vi "Loop.vi"(0 "Input parameters":T2={"Measurement type"=enum."Debug", "Sensor type"=enum."HPK_8in_256", "Identifier"="test.txt", "Open after execution?"=FALSE, "Plot after execution?"=FALSE, "Display channel"=0, "Voltage Delay (s)"=0.5, "Switch Delay (s)"=0.01, "VISA resource name source"="", "VISA resource name DMM"="", "VISA resource name LCR"="", "Compliance  Level (A)"=10.0, "Voltage Limit (V)"=1000.0, "Data storage location"="", "Scan voltages"="", "Use source as DMM?"=FALSE, "LCR signal frequenzy (Hz)"=10.0, "DMM device"=enum."Keithley2001", "Sampling number"=1, "Use env. sensors on"=enum."Sensirion sht1x/7x", "Switchboard Handle"=0, "Use Switchboard"=FALSE, "LCR signal voltage (V)"=10000.0, "Repeat"=1, "Scan voltages IV"="", "Scan voltages CV"="", "Hex pad numbers?"=FALSE, "Set measurement type"=enum."Debug", "Custom pad scan"="", "IV voltage Delay (s)"=0.5, "CV voltage Delay (s)"=0.5, "Needle measurement?"=FALSE, "Comments"="test.txt", "LCR signal frequenzy (kHz)"=10.0, "Compliance  Level (uA)"=10.0, "Open Correction Array"=array2304x3[6912 elements], "Current set voltage"=0.0, "Last set voltage"=0.0, "Current channel"=0, "Last OpenCorrection index"=-1, "Total curr/vltg every x steps"=10, "Current channel iteration"=0, "No CV corrections"=FALSE, "Mapfile"="", "Corrfile"="", "Invert polarity"=FALSE} {"Last set voltage" format="%#_13g"; "Current set voltage" format="%#_13g"; "CV voltage Delay (s)" format="%#_13g"; "IV voltage Delay (s)" format="%#_13g"; "Voltage Limit (V)" format="%#_13g"; "Voltage Delay (s)" format="%#_13g"; "Switch Delay (s)" format="%#_13g"}, 5 "Dynamic data":T4, 7 "Front_panel_refs":T1, 11 "error in (no error)":errorcluster, 12 "Environmental data":T3) -> (4 "Input parameters out":T2={"Measurement type"=enum."Debug", "Sensor type"=enum."HPK_8in_256", "Identifier"="test.txt", "Open after execution?"=FALSE, "Plot after execution?"=FALSE, "Display channel"=0, "Voltage Delay (s)"=0.5, "Switch Delay (s)"=0.01, "VISA resource name source"="", "VISA resource name DMM"="", "VISA resource name LCR"="", "Compliance  Level (A)"=10.0, "Voltage Limit (V)"=1000.0, "Data storage location"="", "Scan voltages"="", "Use source as DMM?"=FALSE, "LCR signal frequenzy (Hz)"=10.0, "DMM device"=enum."Keithley2001", "Sampling number"=1, "Use env. sensors on"=enum."Sensirion sht1x/7x", "Switchboard Handle"=0, "Use Switchboard"=FALSE, "LCR signal voltage (V)"=10000.0, "Repeat"=1, "Scan voltages IV"="", "Scan voltages CV"="", "Hex pad numbers?"=FALSE, "Set measurement type"=enum."Debug", "Custom pad scan"="", "IV voltage Delay (s)"=0.5, "CV voltage Delay (s)"=0.5, "Needle measurement?"=FALSE, "Comments"="test.txt", "LCR signal frequenzy (kHz)"=10.0, "Compliance  Level (uA)"=10.0, "Open Correction Array"=array2304x3[6912 elements], "Current set voltage"=0.0, "Last set voltage"=0.0, "Current channel"=0, "Last OpenCorrection index"=-1, "Total curr/vltg every x steps"=10, "Current channel iteration"=0, "No CV corrections"=FALSE, "Mapfile"="", "Corrfile"="", "Invert polarity"=FALSE} {"Last set voltage" format="%#_13g"; "Current set voltage" format="%#_13g"; "CV voltage Delay (s)" format="%#_13g"; "IV voltage Delay (s)" format="%#_13g"; "Voltage Limit (V)" format="%#_13g"; "Voltage Delay (s)" format="%#_13g"; "Switch Delay (s)" format="%#_13g"}, 6 "Dynamic data out":T4, 8 "Front_panel_refs out":T1, 15 "error out":errorcluster)   [LabVIEW 2016]
uses:
  Input_parameters.ctl
  Dynamic_data.ctl
  <extravilib>/ChannelInstances/Tag-t'Env_data.ctl'/))Channel.ctl
  Env_data.ctl
  Front_panel_refs.ctl
  Live_data.ctl
  <extravilib>/ChannelInstances/Tag-t'Env_data.ctl'/Read With Abort.vi
  <extravilib>/ChannelInstances/Tag-t'Env_data.ctl'/Endpoint.vi
  <extravilib>/ChannelInstances/Tag-t'Env_data.ctl'.lvlib
panel:
  out "Input parameters display":T2={"Measurement type"=enum."Debug", "Sensor type"=enum."HPK_8in_256", "Identifier"="test.txt", "Open after execution?"=FALSE, "Plot after execution?"=FALSE, "Display channel"=0, "Voltage Delay (s)"=0.5, "Switch Delay (s)"=0.01, "VISA resource name source"="", "VISA resource name DMM"="", "VISA resource name LCR"="", "Compliance  Level (A)"=10.0, "Voltage Limit (V)"=1000.0, "Data storage location"="", "Scan voltages"="", "Use source as DMM?"=FALSE, "LCR signal frequenzy (Hz)"=10.0, "DMM device"=enum."Keithley2001", "Sampling number"=1, "Use env. sensors on"=enum."Sensirion sht1x/7x", "Switchboard Handle"=0, "Use Switchboard"=FALSE, "LCR signal voltage (V)"=10000.0, "Repeat"=1, "Scan voltages IV"="", "Scan voltages CV"="", "Hex pad numbers?"=FALSE, "Set measurement type"=enum."Debug", "Custom pad scan"="", "IV voltage Delay (s)"=0.5, "CV voltage Delay (s)"=0.5, "Needle measurement?"=FALSE, "Comments"="test.txt", "LCR signal frequenzy (kHz)"=10.0, "Compliance  Level (uA)"=10.0, "Open Correction Array"=array2304x3[6912 elements], "Current set voltage"=0.0, "Last set voltage"=0.0, "Current channel"=0, "Last OpenCorrection index"=-1, "Total curr/vltg every x steps"=10, "Current channel iteration"=0, "No CV corrections"=FALSE, "Mapfile"="", "Corrfile"="", "Invert polarity"=FALSE} {"Last set voltage" format="%#_13g"; "Current set voltage" format="%#_13g"; "CV voltage Delay (s)" format="%#_13g"; "IV voltage Delay (s)" format="%#_13g"; "Voltage Limit (V)" format="%#_13g"; "Voltage Delay (s)" format="%#_13g"; "Switch Delay (s)" format="%#_13g"}
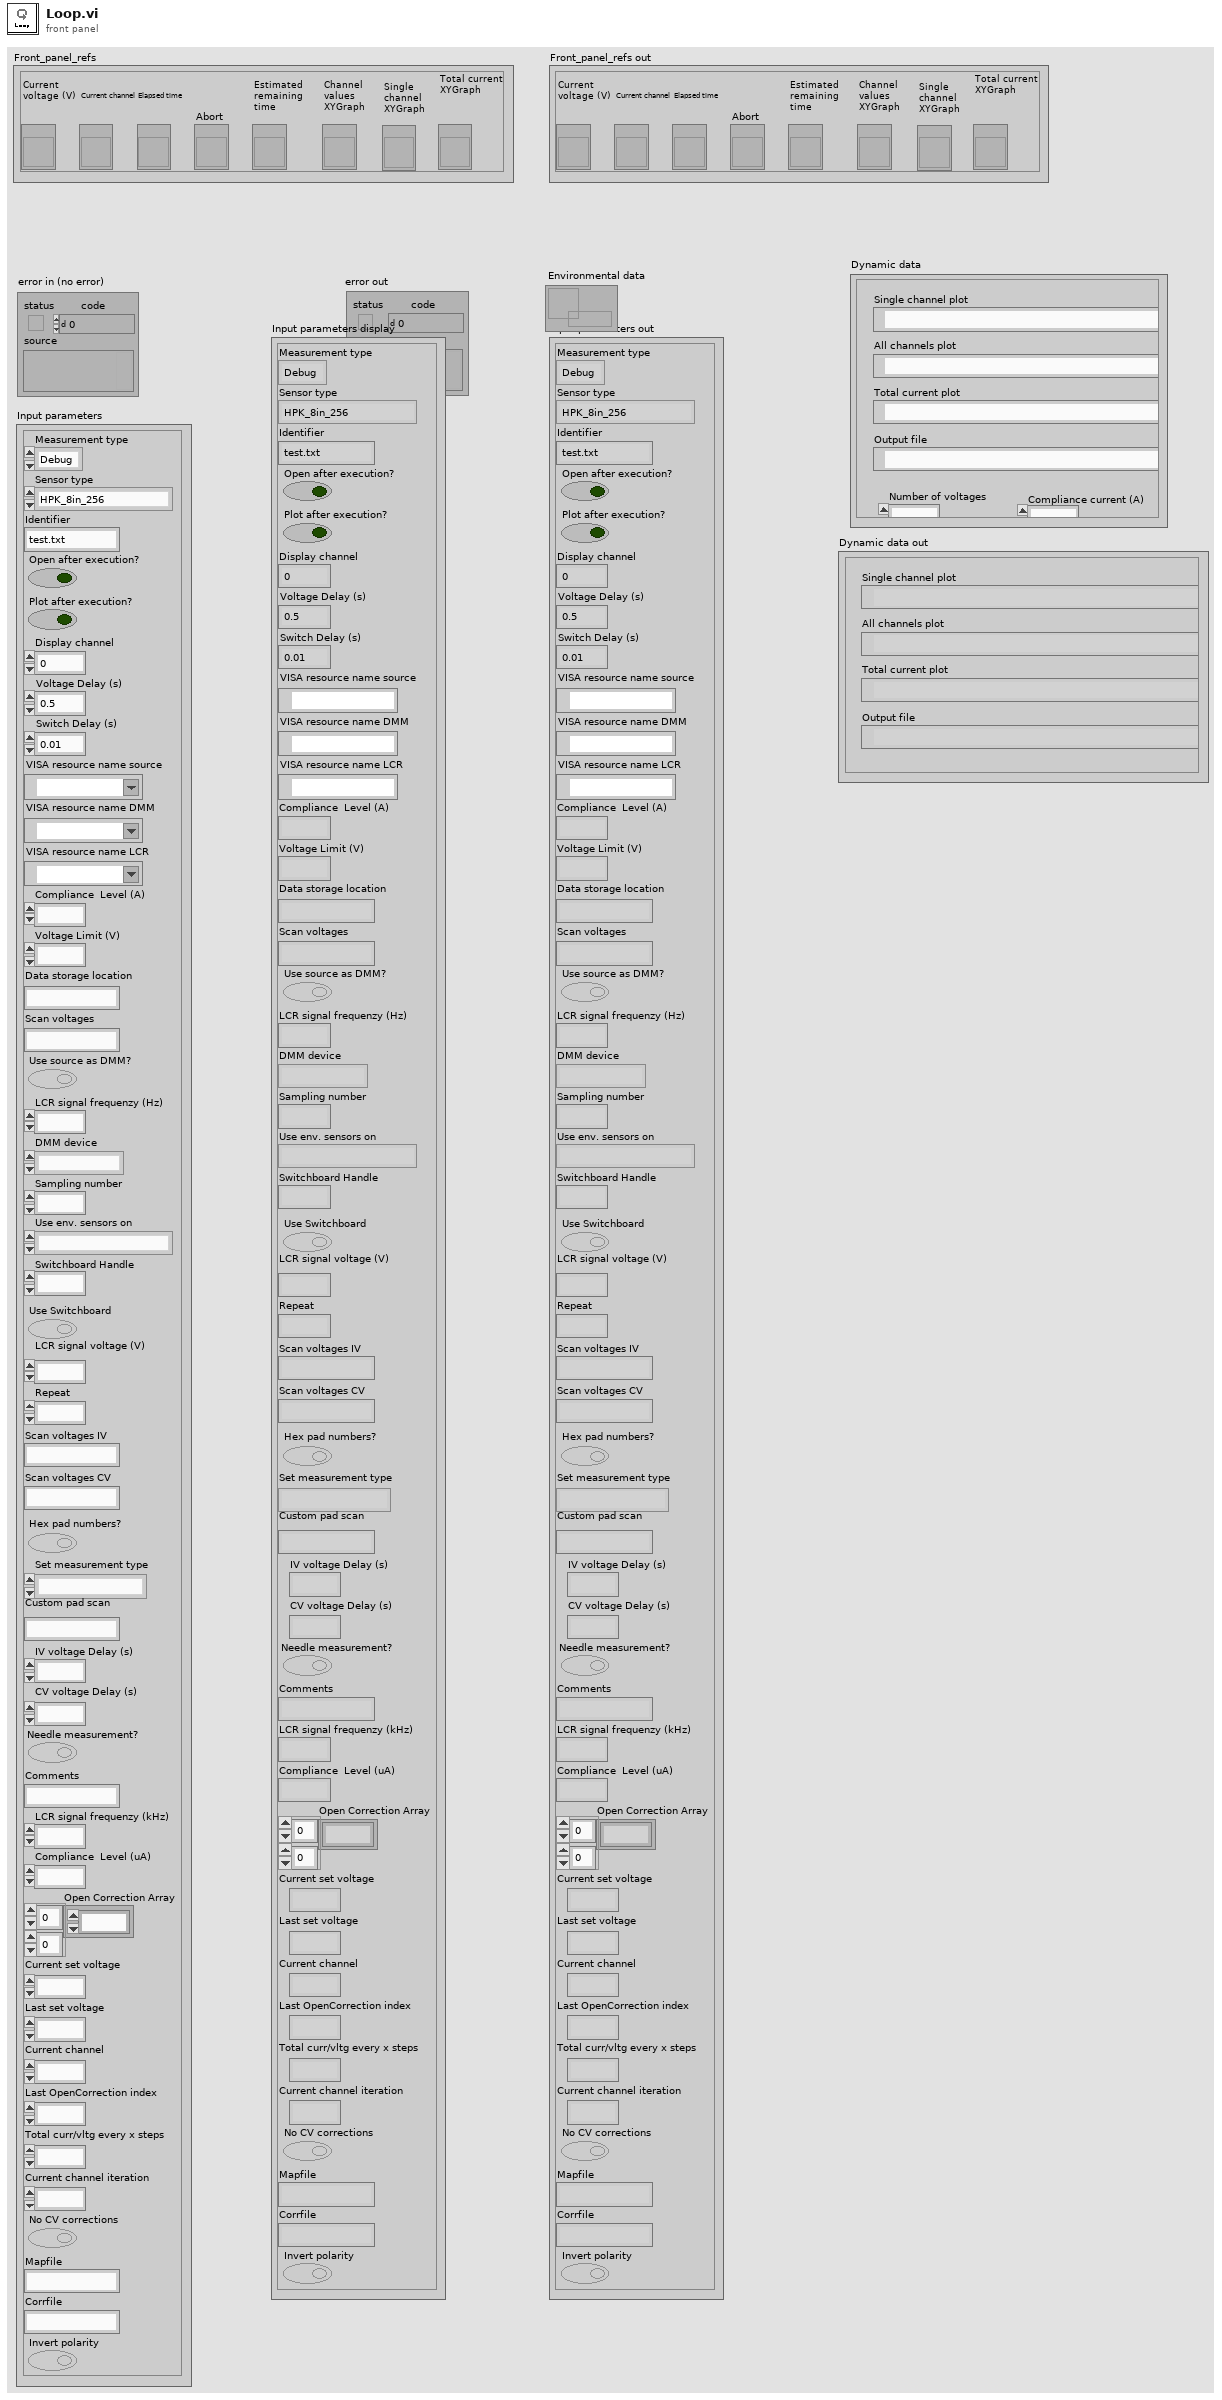
[diagram p1: front panel]
types:
  T1 = typedef "Front_panel_refs.ctl" = cluster{"Current voltage (V)":refnum<vi>, "Elapsed time":refnum<vi>, "Current channel":refnum<vi>, "Abort":refnum<vi>, "Estimated remaining time":refnum<vi>, "Channel values XYGraph":refnum<vi>, "Single channel XYGraph":refnum<vi>, "Total current XYGraph":refnum<vi>}
  T2 = typedef "Input_parameters.ctl" = cluster{"Measurement type":enum16{"IV", "CV", "Debug", "Test_contact"}, "Sensor type":enum16{"HPK_6in_135", "HPK_8in_256", "IFX_8in_256", "Diode", "HPK_6in_256", "Full matrix"}, "Identifier":string, "Open after execution?":bool, "Plot after execution?":bool, "Display channel":i32, "Voltage Delay (s)":dbl, "Switch Delay (s)":dbl, "VISA resource name source":refnum<visa-resource-name>, "VISA resource name DMM":refnum<visa-resource-name>, "VISA resource name LCR":refnum<visa-resource-name>, "Compliance  Level (A)":dbl, "Voltage Limit (V)":dbl, "Data storage location":string, "Scan voltages":string, "Use source as DMM?":bool, "LCR signal frequenzy (Hz)":dbl, "DMM device":enum16{"Keithley2001", "Keithley2450", "Keithley2410", "Keithley6487"}, "Sampling number":i32, "Use env. sensors on":enum16{"Sensirion sht1x/7x", "Switch Matrix", "Probecard"}, "Switchboard Handle":u32, "Use Switchboard":bool, "LCR signal voltage (V)":dbl, "Repeat":i32, "Scan voltages IV":string, "Scan voltages CV":string, "Hex pad numbers?":bool, "Set measurement type":enum16{"IV", "CV", "Debug", "Test_contact", "IV+CV"}, "Custom pad scan":string, "IV voltage Delay (s)":dbl, "CV voltage Delay (s)":dbl, "Needle measurement?":bool, "Comments":string, "LCR signal frequenzy (kHz)":dbl, "Compliance  Level (uA)":dbl, "Open Correction Array":dbl[][], "Current set voltage":dbl, "Last set voltage":dbl, "Current channel":i32, "Last OpenCorrection index":i32, "Total curr/vltg every x steps":i32, "Current channel iteration":i32, "No CV corrections":bool, "Mapfile":string, "Corrfile":string, "Invert polarity":bool}
  T3 = typedef "Tag-t'Env_data.ctl'.lvlib/))Channel.ctl" = refnum<queue>
  T4 = typedef "Dynamic_data.ctl" = cluster{"Output file":path, "Y-label text":string, "Current set voltage":dbl, "Set voltage column":dbl[], "Pad number column":dbl[], "Data  column":dbl[], "Number of voltages":i32, "Compliance current (A)":dbl, "Geofile":string, "Peak voltage":dbl, "Hex PDF file":string, "Voltage array":dbl[], "Total current column":dbl[], "Timestamp column":dbl[], "Data name":string, "Data unit":string, "2nd data column":dbl[], "2nd data name":string, "2nd data unit":string, "3rd data column":dbl[], "4th data column":dbl[], "3rd data name":string, "3rd data unit":string, "4th data name":string, "4th data unit":string, "Actual voltage column":dbl[], "2nd Y-label text":string, "Single channel plot":path, "Temperature column":dbl[], "Humidity column":dbl[], "Channel switch array":i32[], "1st single plot name":string, "2nd single plot name":string, "All channels plot":path, "HexPlot command":string, "Custom channel array":i32[], "Data  error column":dbl[], "2nd data  error column":dbl[], "3rd data error column":dbl[], "4th data  error column":dbl[], "Total current plot":path, "5th data column":dbl[], "5th data  error column":dbl[], "6th data column":dbl[], "6th data  error column":dbl[], "5th data name":string, "5th data unit":string, "6th data name":string, "6th data unit":string, "HexPlot matrix command":string}
  T5 = typedef "Live_data.ctl" = cluster{"Actual voltage":dbl, "Total current":dbl, "Data":dbl, "Data error":dbl, "2nd data":dbl, "2nd data error":dbl, "3rd data":dbl, "3rd data error":dbl, "4th data":dbl, "4th data error":dbl, "6th data error":dbl, "6th data":dbl, "5th data error":dbl, "5th data":dbl}
  T6 = enum16{"Sensirion sht1x/7x", "Switch Matrix", "Probecard"}
  T7 = typedef "Env_data.ctl" = cluster{"Temp. Sensirion":dbl, "Hum. Sensirion":dbl, "Temp. Switch Matrix":dbl, "Hum. Switch Matrix":dbl, "Temp. Probecard":dbl, "Hum. Probecard":dbl}
  T8 = cluster{"XY Graph out":cluster{"Array":dbl[], "Array":dbl[]}[], "XY Graph out":cluster{"Array":dbl[], "Array":dbl[]}[]}
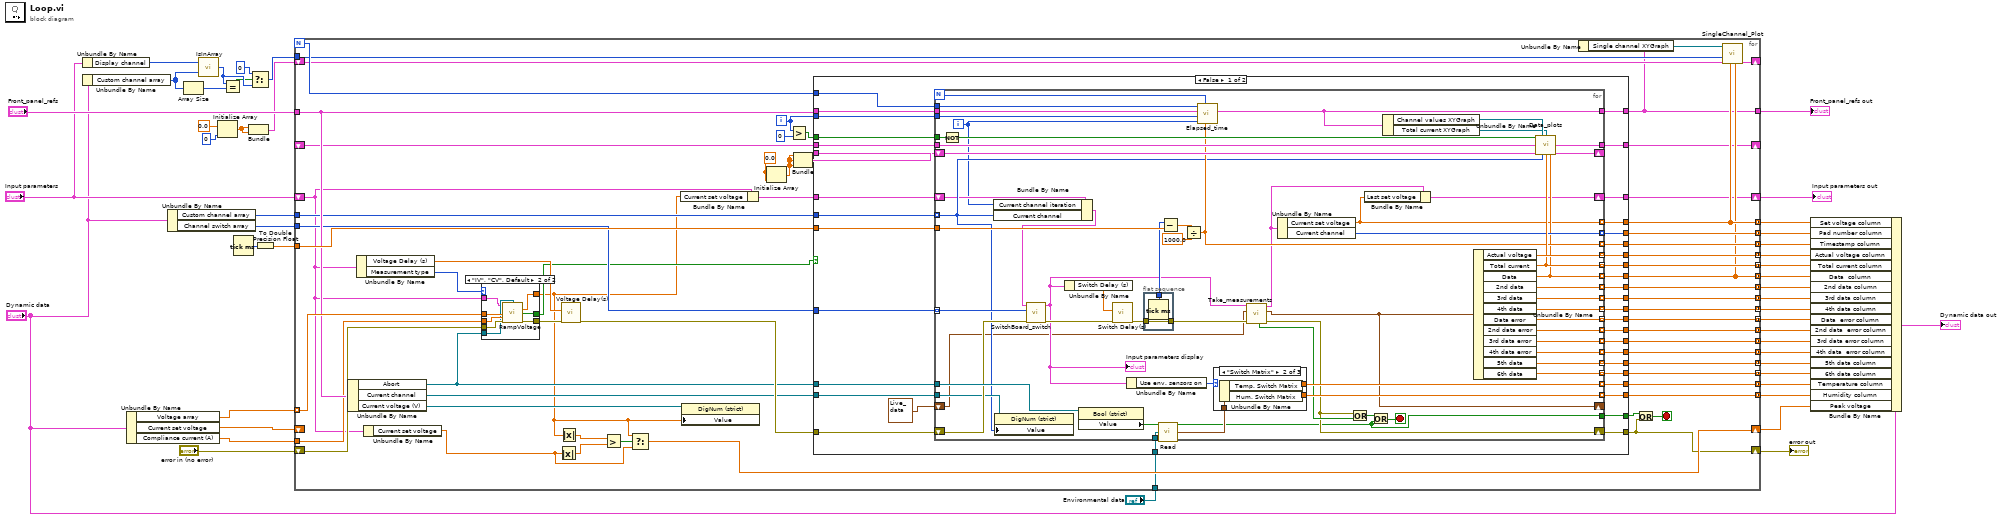
[diagram p0: block diagram]
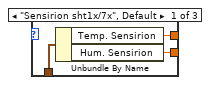
[diagram p2: hidden frame]
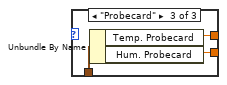
[diagram p3: hidden frame]
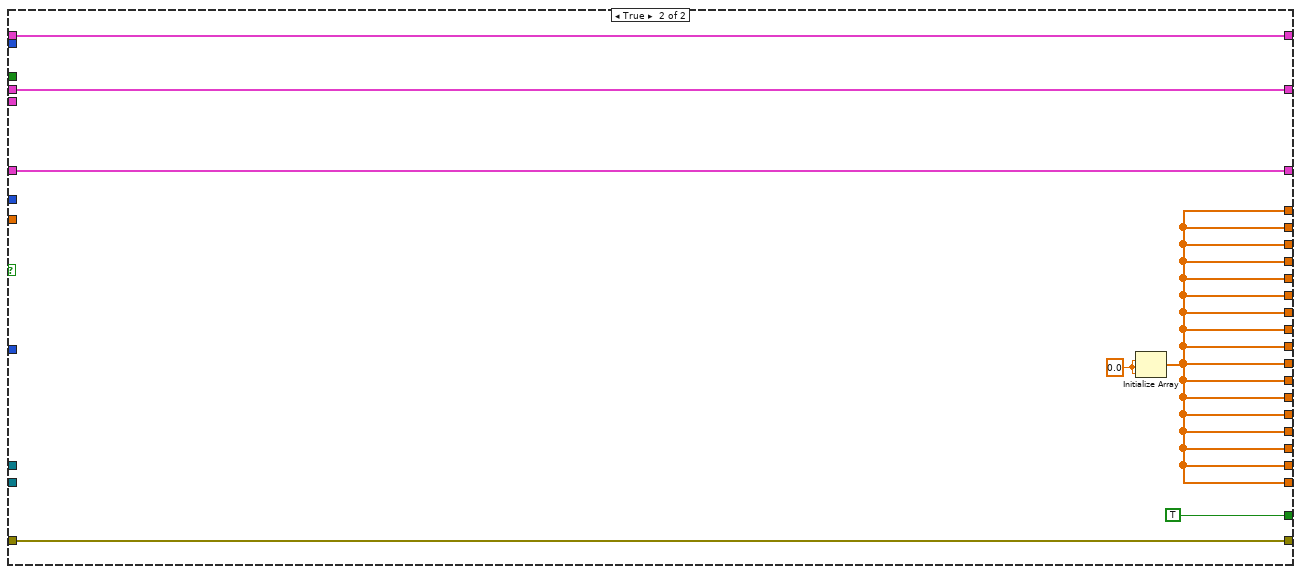
[diagram p4: hidden frame]
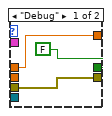
[diagram p5: hidden frame]
diagram:
  n1 = Unbundle By Name("Input parameters") -> ("Display channel"=w23:i32)
  n2 = Unbundle By Name("Dynamic data") -> ("Custom channel array"=w22:i32[])
  n3 = Unbundle By Name("Dynamic data") -> ("Voltage array"=w24:dbl[], "Current set voltage"=w9:dbl, "Compliance current (A)"=w8:dbl)
  n4 = Unbundle By Name("Dynamic data") -> ("Custom channel array"=w15:i32[], "Channel switch array"=w14:i32[])
  n5 = Array Size(array=w22) -> (size(s)=w18:i32)
  n6 = call "IsInArray.vi"("Array"=w22, "Numeric"=w23) -> ("Position"=w20:i32)
  n7 = Initialize Array(0.0 ("Secondary Parameter"), 0 ("dimension size")) -> (w11:dbl[])
  n8 = Equal?(x=w20, y=w18) -> (x = y?=w19:bool)
  n9 = Tick Count (ms)() -> (millisecond timer value=w26:u32)
  n10 = Bundle(w11, w11) -> (w10:cluster{dbl[], dbl[]})  [unwired: 1 in]
  n11 = Select(t=0, s=w19, f=w20) -> (s? t:f=w16:i32)
  n12 = To Double Precision Float(number=w26) -> (double precision float=w25:dbl)
  n13 = for {
    N -> [w89]
    tunnel: w24 -> [w97] mode=indexing
    tunnel: [w81] -> w5 mode=concatenating
    tunnel: [w80] -> w45 mode=concatenating
    tunnel: [w103] -> w4 mode=concatenating
    shift-right: [w57] -> w42
    shift-left: "error in (no error)" -> [w102]
    shift-right: [w73] -> w43
    shift-left: "Input parameters" -> [w46]
    tunnel: w25 -> [w93]
    shift-right: [w98] -> w37
    shift-left: w9 -> [_]
    tunnel: [w94] -> w6 mode=concatenating
    tunnel: [w92] -> w7 mode=concatenating
    tunnel: [w91] -> w41 mode=concatenating
    tunnel: [w88] -> w40 mode=concatenating
    tunnel: [w87] -> w39 mode=concatenating
    tunnel: [w86] -> w38 mode=concatenating
    tunnel: [w85] -> w36 mode=concatenating
    tunnel: [w84] -> w35 mode=concatenating
    tunnel: "Environmental data" -> [w83]
    tunnel: [w79] -> w31 mode=concatenating
    tunnel: [w78] -> w30 mode=concatenating
    tunnel: [w77] -> w29 mode=concatenating
    tunnel: [w76] -> w28 mode=concatenating
    tunnel: "Front_panel_refs" -> [w74]
    tunnel: w16 -> [w60]
    tunnel: w8 -> [w69]
    tunnel: w15 -> [w68]
    tunnel: w14 -> [w67]
    shift-right: [w64] -> _
    shift-left: _ -> [w63]
    shift-right: [w61] -> _
    shift-left: w10 -> [w62]
    tunnel: [w55] -> w3 mode=concatenating
    tunnel: [w54] -> w2 mode=concatenating
    tunnel: [w48] -> w1
    i -> [w90]
    stop <- w99 stop-if-true
    w82 = 0.0 ("dimension size")
    n14 = Unbundle By Name(w74) -> ("Abort"=w75:refnum<vi>, "Current channel"=w71:refnum<vi>, "Current voltage (V)"=w72:refnum<vi>)
    n15 = Unbundle By Name(w46) -> ("Voltage Delay (s)"=w70:dbl, "Measurement type"=w96:enum16{"IV", "CV", "Debug", "Test_contact"})
    n16 = Unbundle By Name(w46) -> ("Current set voltage"=w49:dbl)
    n17 = case shown="\"IV\", \"CV\", Default" w96 {
      tunnel: w97 -> [w220 w227]
      tunnel: w102 -> [w221 w228]
      tunnel: [w221 w229] -> w101
      tunnel: w69 -> [_ w226]
      tunnel: [w220 w225] -> w50
      tunnel: w75 -> [_ w224]
      tunnel: [FALSE ("Aborted?") w223] -> w56
      tunnel: w46 -> [_ w222]
      frame "Debug" {
      }
      frame "IV", "CV", Default {
        n18 = call "RampVoltage.vi"("Input parameters"=w222, "Stop"=w224, "Target voltage (V)"=w227, "Compliance Current (A)"=w226, "error in (no error)"=w228) -> ("Current voltage out (V)"=w225:dbl, "Aborted?"=w223:bool, "error out"=w229:errorcluster)  [unwired: 7 in, 1 out]
      }
    }
    n19 = Absolute Value(x=w49) -> (abs(x)=w51:dbl)
    n20 = Absolute Value(x=w50) -> (abs(x)=w52:dbl)
    n21 = call "Voltage Delay(s)"("error in (no error)"=w101, "Delay Time (s)"=w70) -> ("error out"=w95:errorcluster)  [unwired: 9 in]
    n22 = Greater?(x=w52, y=w51) -> (0:w53:bool)
    n23 = Select(t=w50, s=w53, f=w49) -> (s? t:f=w98:dbl)
    n24 = Bundle By Name(cluster=w46, "Current set voltage"=w50) -> (w59:T2)
    n25 = property class="DigNum (strict)"(reference=w72, "Value"=w50) -> ()  [unwired: 1 in, 2 out]
    n26 = Initialize Array(w82, w82) -> (w66:dbl[])
    n27 = Greater?(x=w90, y=0) -> (0:w100:bool)
    n28 = Bundle(w66, w66, w66) -> (w65:cluster{dbl[], dbl[], dbl[]})  [unwired: 1 in]
    n29 = case shown="False" w56 {
      tunnel: [w141 w213] -> w103
      tunnel: w100 -> [w140 _]
      tunnel: w95 -> [w139 w216]
      tunnel: [w138 w213] -> w94
      tunnel: w93 -> [w137 _]
      tunnel: [w136 w213] -> w92
      tunnel: [w135 w213] -> w91
      tunnel: w90 -> [w134 _]
      tunnel: w89 -> [w133 _]
      tunnel: [w132 w213] -> w88
      tunnel: [w131 w213] -> w87
      tunnel: [w130 w213] -> w86
      tunnel: [w129 w213] -> w85
      tunnel: [w128 w213] -> w84
      tunnel: w83 -> [w127 _]
      tunnel: [w126 w213] -> w81
      tunnel: [w125 w213] -> w80
      tunnel: [w124 w213] -> w79
      tunnel: [w123 w213] -> w78
      tunnel: [w122 w213] -> w77
      tunnel: [w121 w213] -> w76
      tunnel: w75 -> [w120 _]
      tunnel: w74 -> [w119 w212]
      tunnel: [w118 w218] -> w73
      tunnel: w71 -> [w117 _]
      tunnel: w68 -> [w116 _]
      tunnel: w67 -> [w115 _]
      tunnel: w65 -> [w114 _]
      tunnel: [w113 w217] -> w64
      tunnel: w63 -> [w112 w217]
      tunnel: w59 -> [w111 w218]
      tunnel: [w110 TRUE ("Value")] -> w58
      tunnel: [w109 w216] -> w57
      tunnel: [w108 w213] -> w54
      tunnel: [w107 w213] -> w55
      tunnel: [w105 w212] -> w48
      frame False {
        n30 = for {
          N -> [w164]
          tunnel: w115 -> [w185] mode=indexing
          tunnel: [w161] -> w141 mode=indexing
          tunnel: [w158] -> w125 mode=indexing
          tunnel: [w148] -> w126 mode=indexing
          shift-right: [w156] -> w109
          shift-left: w139 -> [w187]
          tunnel: w140 -> [w179]
          tunnel: [w154] -> w110
          tunnel: w120 -> [w200]
          tunnel: [w167] -> w138 mode=indexing
          tunnel: w137 -> [w199]
          tunnel: [w165] -> w136 mode=indexing
          tunnel: [w178] -> w135 mode=indexing
          tunnel: w134 -> [w172]
          tunnel: w133 -> [w163]
          tunnel: [w194] -> w132 mode=indexing
          tunnel: [w193] -> w131 mode=indexing
          tunnel: [w192] -> w130 mode=indexing
          tunnel: [w190] -> w129 mode=indexing
          tunnel: [w189] -> w128 mode=indexing
          tunnel: w127 -> [w188]
          tunnel: w116 -> [w162] mode=indexing
          tunnel: [w183] -> w124 mode=indexing
          tunnel: [w182] -> w123 mode=indexing
          tunnel: [w181] -> w122 mode=indexing
          tunnel: [w180] -> w121 mode=indexing
          tunnel: w117 -> [w175]
          tunnel: w119 -> [w171]
          shift-right: [w170] -> _
          shift-left: w114 -> [w166]
          tunnel: [w168] -> w113
          tunnel: w112 -> [w169]
          shift-right: [w150] -> w118
          shift-left: w111 -> [w160]
          tunnel: [w152] -> w108 mode=indexing
          tunnel: [w151] -> w107 mode=indexing
          shift-right: [w147] -> _
          shift-left: T5 {"Actual voltage"=0.0, "Total current"=0.0, "Data"=0.0, "Data error"=0.0, "2nd data"=0.0, "2nd data error"=0.0, "3rd data"=0.0, "3rd data error"=0.0, "4th data"=0.0, "4th data error"=0.0, "6th data error"=0.0, "6th data"=0.0, "5th data error"=0.0, "5th data"=0.0} ("Live data out") -> [w146]
          tunnel: [w144] -> w105
          i -> [w145]
          stop <- w153 stop-if-true
          n31 = Not(x=w179) -> (.not. x?=w177:bool)
          n32 = Bundle By Name(cluster=w160, "Current channel iteration"=w145, "Current channel"=w162) -> (w159:T2)
          n33 = property on="Property Node" class="DigNum (strict)"(reference=w175, "Value"=w162) -> ()  [unwired: 1 in, 2 out]
          n34 = call "SwitchBoard_switch.vi"("error in"=w187, "Channel"=w185, "Input parameters in"=w159) -> ("error out"=w186:errorcluster, "Input parameters out"=w173:T2)  [unwired: 7 in]
          "Input parameters display" <- w173
          n35 = Unbundle By Name(w173) -> ("Switch Delay (s)"=w176:dbl)
          n36 = property class="Bool (strict)"(reference=w200) -> ("Value"=w154:bool)  [unwired: 1 in, 2 out]
          n37 = call "Switch Delay(s)"("error in (no error)"=w186, "Delay Time (s)"=w176) -> ("error out"=w196:errorcluster)  [unwired: 9 in]
          n38 = Unbundle By Name(w173) -> ("Use env. sensors on"=w184:T6)
          n39 = flat-sequence {
            tunnel: [w211] -> w197
            tunnel: w196 -> [w210]
            tunnel: [w210] -> w195
            frame #0 {
              n40 = Tick Count (ms)() -> (millisecond timer value=w211:u32)
            }
          }
          n41 = call <extravilib>:"Read.vi"("channel"=w188) -> ("element"=w191:T7)  [unwired: 1 in, 1 out]
          n42 = Subtract(x=w197, y=w199) -> (x-y=w174:dbl)
          n43 = Divide(x=w174, y=1000.0) -> (x/y=w165:dbl)
          n44 = call "Elapsed_time.vi"("Elapsed time (s)"=w165, "Inner N"=w164, "Inner i"=w145, "Outer i"=w172, "Front_panel_refs"=w171, "Outer N"=w163) -> ("Front_panel_refs out"=w144:T1)  [unwired: 5 in]
          n45 = case shown="\"Switch Matrix\"" w184 {
            tunnel: w191 -> [w203 w206 w209]
            tunnel: [w202 w204 w207] -> w190
            tunnel: [w201 w205 w208] -> w189
            frame "Sensirion sht1x/7x", Default {
              n46 = Unbundle By Name(w203) -> ("Temp. Sensirion"=w202:dbl, "Hum. Sensirion"=w201:dbl)
            }
            frame "Switch Matrix" {
              n47 = Unbundle By Name(w206) -> ("Temp. Switch Matrix"=w204:dbl, "Hum. Switch Matrix"=w205:dbl)
            }
            frame "Probecard" {
              n48 = Unbundle By Name(w209) -> ("Temp. Probecard"=w207:dbl, "Hum. Probecard"=w208:dbl)
            }
          }
          n49 = call "Take_measurements.vi"("error in (no error)"=w195, "Live data in"=w146, "Input parameters"=w173) -> ("error out"=w156:errorcluster, "Live data out"=w147:T5, "Input parameters out"=w149:T2, "Compliance reached?"=w157:bool)  [unwired: 5 in]
          n50 = Unbundle By Name(w149) -> ("Current set voltage"=w148:dbl, "Current channel"=w161:i32)
          n51 = Or(x=w156, y=w157) -> (x .or. y?=w155:bool)
          n52 = Bundle By Name(cluster=w149, "Last set voltage"=w148) -> (w150:T2)
          n53 = Or(x=w155, y=w154) -> (x .or. y?=w153:bool)
          n54 = Unbundle By Name(w144) -> ("Channel values XYGraph"=w143:refnum<vi>, "Total current XYGraph"=w142:refnum<vi>)
          n55 = Unbundle By Name(w147) -> ("Actual voltage"=w192:dbl, "Total current"=w167:dbl, "Data"=w158:dbl, "2nd data"=w178:dbl, "3rd data"=w194:dbl, "4th data"=w193:dbl, "Data error"=w183:dbl, "2nd data error"=w182:dbl, "3rd data error"=w181:dbl, "4th data error"=w180:dbl, "5th data"=w152:dbl, "6th data"=w151:dbl)
          n56 = call "Data_plots.vi"("Is first?"=w177, "Channels"=w143, 2:"Total current"=w142, "Plot cluster"=w169, "Cluster"=w166, "Custom channel"=w162, 13:"Total current"=w167, "Data"=w158) -> ("Plot cluster out"=w168:T8, "Cluster out"=w170:cluster{dbl[], dbl[], dbl[]})  [unwired: 6 in]
        }
      }
      frame True {
        w214 = 0.0 ("dimension size")
        n57 = Initialize Array(w214, w214) -> (w213:dbl[])
      }
    }
    n58 = Unbundle By Name(w48) -> ("Single channel XYGraph"=w47:refnum<vi>)
    n59 = Or(x=w58, y=w57) -> (x .or. y?=w99:bool)
    n60 = call "SingleChannel_Plot.vi"("Data column"=w80, "Set voltage column"=w81, "Cluster"=w62, "Channel"=w60, "Single channel ref"=w47) -> ("Cluster out"=w61:cluster{dbl[], dbl[]})  [unwired: 6 in]
  }
  "error out" <- w42
  "Input parameters out" <- w43
  "Front_panel_refs out" <- w1
  n61 = Bundle By Name(cluster="Dynamic data", "Set voltage column"=w5, "Pad number column"=w4, "Timestamp column"=w7, "Actual voltage column"=w38, "Total current column"=w6, "Data  column"=w45, "2nd data column"=w41, "3rd data column"=w40, "4th data column"=w39, "Data  error column"=w31, "2nd data  error column"=w30, "3rd data error column"=w29, "4th data  error column"=w28, "5th data column"=w2, "6th data column"=w3, "Temperature column"=w36, "Humidity column"=w35, "Peak voltage"=w37) -> (→"Dynamic data out":T4)
